vi "Preset subsystems.vi"(10 "appended array":bool[](array[boolean]), 11 "Enum":T1(ring)=enum."Low Hatch") -> ()   [LabVIEW 2019]
uses:
  5daef287-ccd4-4bc1-8e60-40fa11514e16.vi
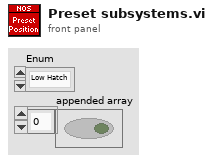
[diagram p1: front panel]
types:
  T1 = enum16{"Pick Up Ball", "Pick Up Hatch", "Shoot Ball", "Shoot Hatch", "Low Ball", "Middle Ball", "High Ball", "High Hatch", "Middle Hatch", "Low Hatch", "Cargo Ball", "Ball Loading Station", "Ball Ground", "Reserve"}
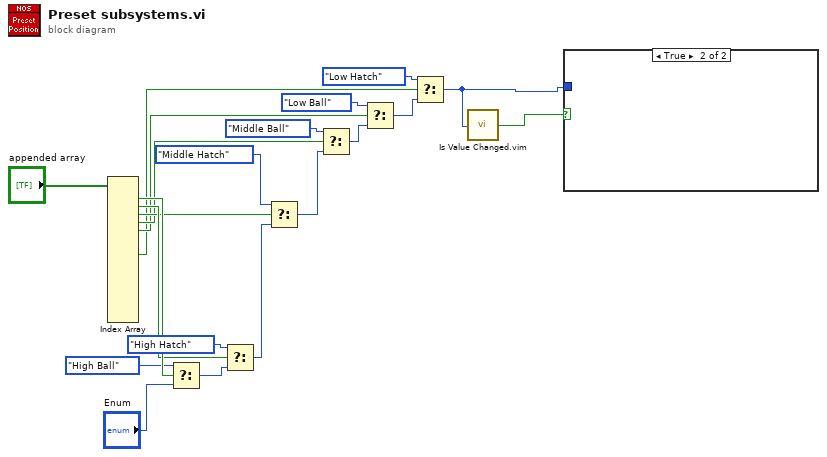
[diagram p0: block diagram]
diagram:
  n1 = Index Array(array="appended array") -> (element #1=w20:bool, element #2=w17:bool, element #3=w16:bool, element #4=w13:bool, element #5=w11:bool, element #8=w3:bool)  [unwired: 16 in, 10 out]
  n2 = Select(t=T1."High Ball" ("Enum 2"), s=w20, f="Enum") -> (s? t:f=w18:T1)
  n3 = Select(t=T1."High Hatch" ("Enum 2"), s=w17, f=w18) -> (s? t:f=w15:T1)
  n4 = Select(t=T1."Middle Hatch" ("Enum 2"), s=w16, f=w15) -> (s? t:f=w14:T1)
  n5 = Select(t=T1."Middle Ball" ("Enum 2"), s=w13, f=w14) -> (s? t:f=w12:T1)
  n6 = Select(t=T1."Low Ball" ("Enum 2"), s=w11, f=w12) -> (s? t:f=w10:T1)
  n7 = Select(t=T1."Low Hatch" ("Enum 2"), s=w3, f=w10) -> (s? t:f=w1:T1)
  n8 = call "Is Value Changed.vim"("value"=w1) -> ("changed or first call?"=w2:bool)
  n9 = case shown="True" w2 {
    tunnel: w1 -> [_ _]
    frame False {
    }
    frame True {
    }
  }
